vi "TriangleCache.vi"(4 "Point3D":T1, 6 "Rotation":T2, 8 "TriangleOperations":T4(ring), 9 "ScaleFac":sgl, 10 "ModelName":string, 11 "TrianglesIn":T3[](array[typedef])) -> (3 "TrianglesOut":T3[](array[typedef]))   [LabVIEW 2014]
uses:
  TypeDefs/TriangleFace.ctl
  TypeDefs/Point3D.ctl
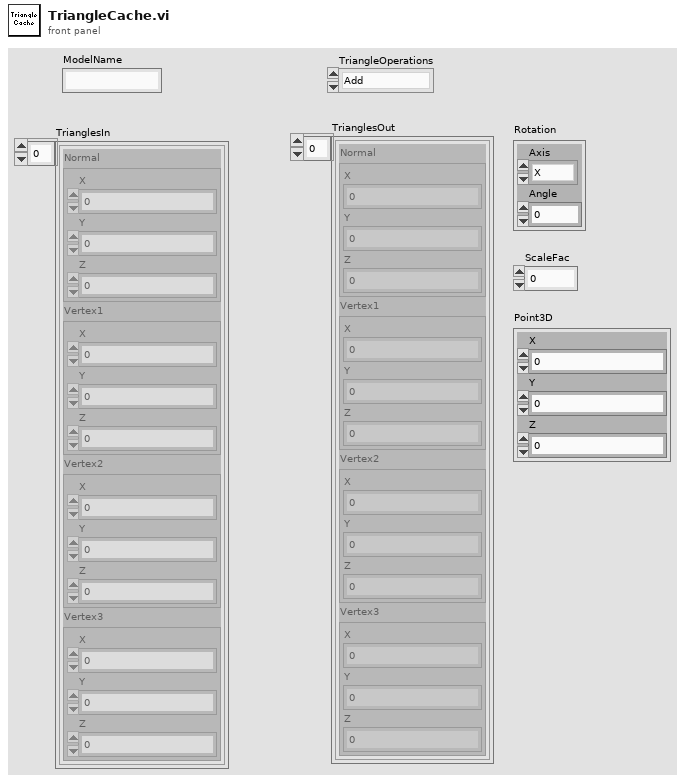
[diagram p1: front panel]
types:
  T1 = typedef "Point3D.ctl" = cluster{"X":sgl, "Y":sgl, "Z":sgl}
  T2 = cluster{"Axis":enum16{"X", "Y", "Z"}, "Angle":sgl}
  T3 = typedef "TriangleFace.ctl" = cluster{"Normal":T1, "Vertex1":T1, "Vertex2":T1, "Vertex3":T1}
  T4 = enum16{"Add", "Get", "Scale", "Rotate", "Translate", "Symmetry", "Clear"}
  T5 = cluster{"ModelName":string, "TrianglesOut":T3[]}[]
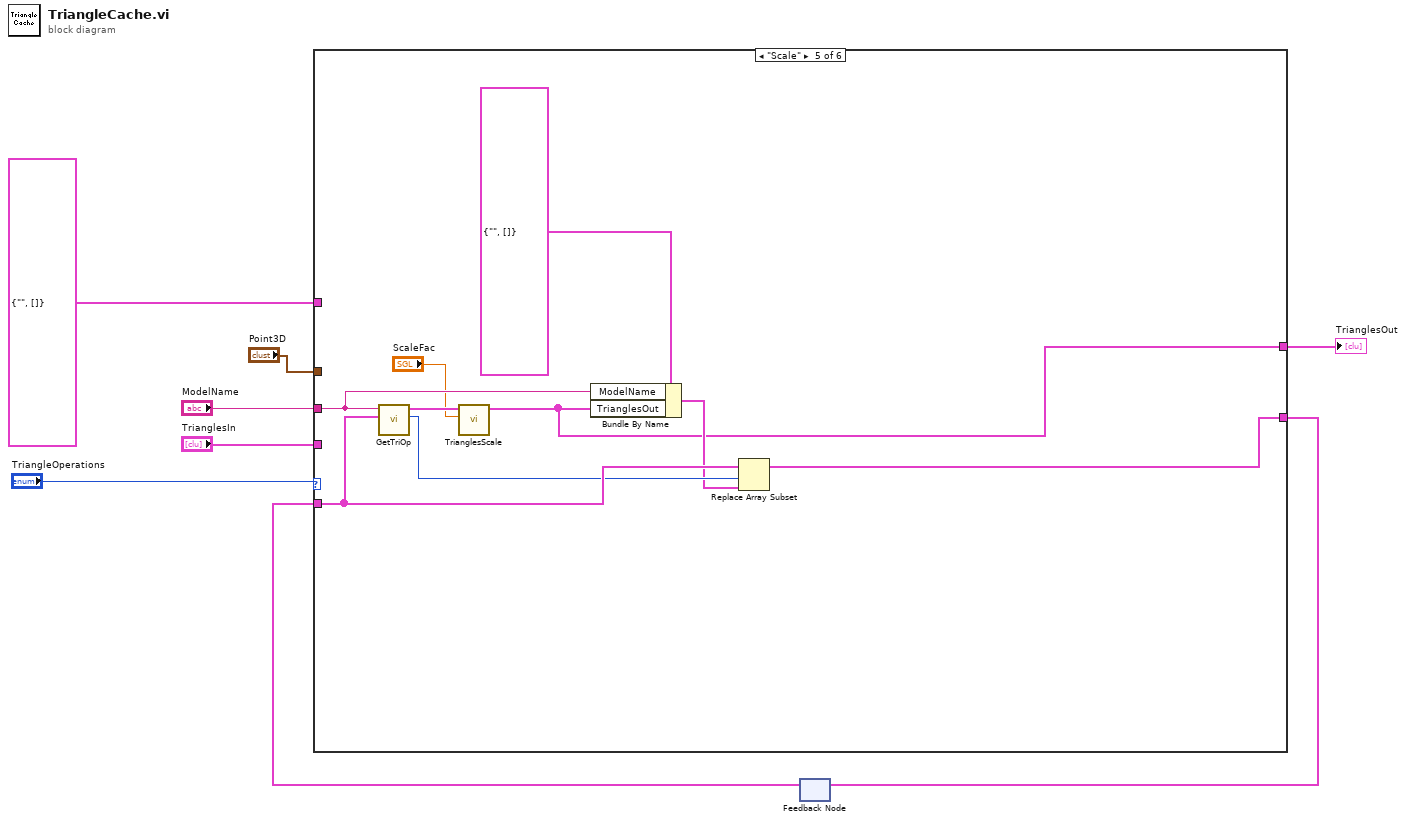
[diagram p0: block diagram]
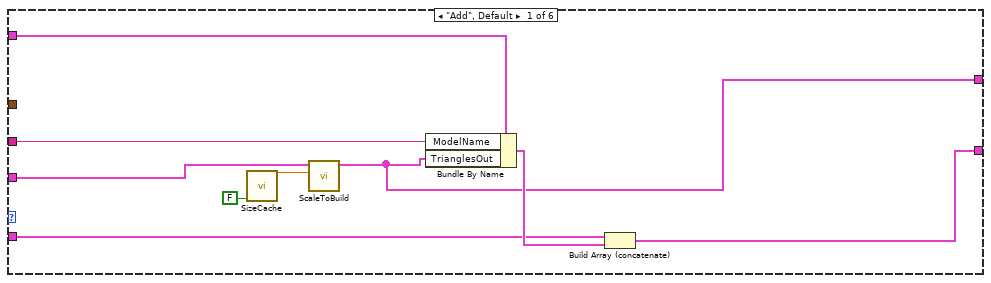
[diagram p2: hidden frame]
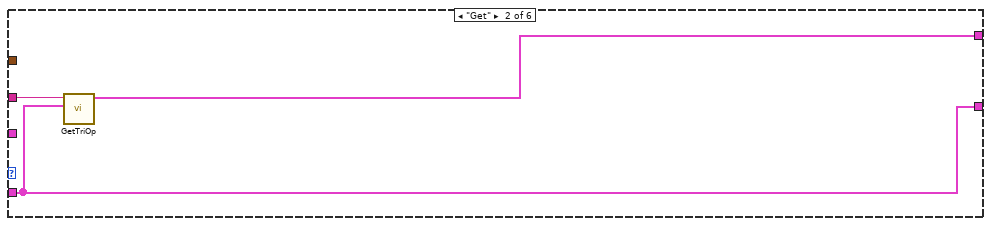
[diagram p3: hidden frame]
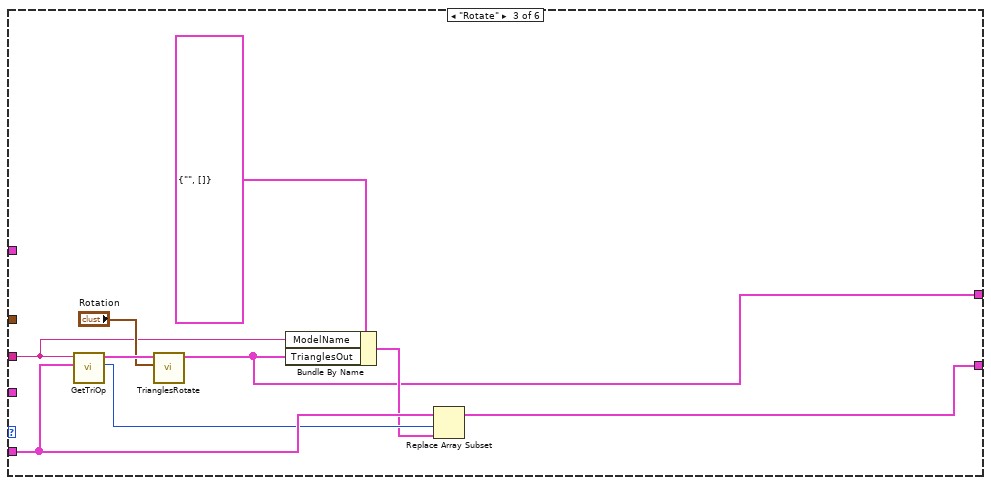
[diagram p4: hidden frame]
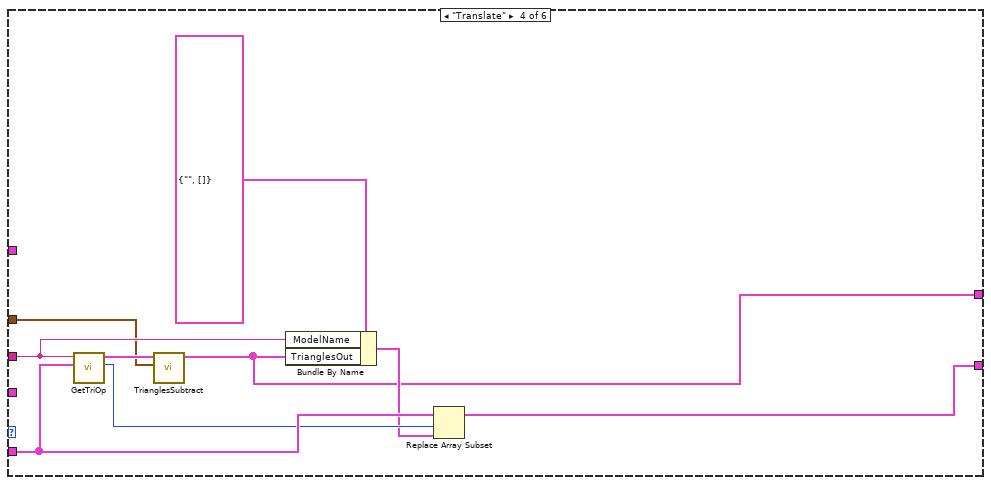
[diagram p5: hidden frame]
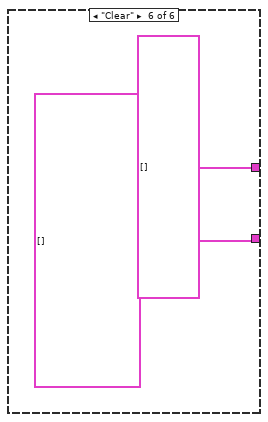
[diagram p6: hidden frame]
diagram:
  n1 = feedback #1() -> (w3:T5)  [unwired: 1 in]
  n2 = case shown="\"Scale\"" "TriangleOperations" {
    tunnel: cluster{"ModelName":string, "TrianglesOut":T3[]} {"ModelName"="", "TrianglesOut"=[]} ("Model") -> [w17 _ _ _ _ _]
    tunnel: "ModelName" -> [w16 w20 w24 w34 w43 _]
    tunnel: "TrianglesIn" -> [w10 _ _ _ _ _]
    tunnel: [w13 w18 w22 w32 w41 T5 []] -> w4
    tunnel: w3 -> [w14 w18 w27 w37 w46 _]
    tunnel: [w9 w19 w21 w31 w40 T3[] [] ("TrianglesOut")] -> w2
    tunnel: "Point3D" -> [_ _ _ w30 _ _]
    frame "Add", Default {
      n3 = call "SizeCache.vi"("Set"=FALSE) -> ("SizeOut"=w11:dbl)  [unwired: 10 in]
      n4 = call "ScaleToBuild.vi"("BuildSize"=w11, "Triangles"=w10) -> ("TrianglesOut"=w9:T3[])  [unwired: 9 in]
      n5 = Bundle By Name(cluster=w17, "ModelName"=w16, "TrianglesOut"=w9) -> (w15:cluster{"ModelName":string, "TrianglesOut":T3[]})
      n6 = Build Array (concatenate)(w14, w15) -> (w13:T5)
    }
    frame "Get" {
      n7 = call "GetTriOp.vi"("Array"=w18, "ModelName"=w20) -> ("TrianglesOut"=w19:T3[])  [unwired: 8 in, 1 out]
    }
    frame "Rotate" {
      n8 = call "GetTriOp.vi"("Array"=w27, "ModelName"=w24) -> ("Index"=w26:i32, "TrianglesOut"=w29:T3[])  [unwired: 8 in]
      n9 = call "TrianglesRotate.vi"("Rotation"="Rotation", "TrianglesIn"=w29) -> ("TrianglesOut"=w21:T3[])  [unwired: 9 in]
      n10 = Bundle By Name(cluster=cluster{"ModelName":string, "TrianglesOut":T3[]} {"ModelName"="", "TrianglesOut"=[]} ("Model"), "ModelName"=w24, "TrianglesOut"=w21) -> (w23:cluster{"ModelName":string, "TrianglesOut":T3[]})
      n11 = Replace Array Subset(array=w27, new element=w23, index=w26) -> (w22:T5)
    }
    frame "Translate" {
      n12 = call "GetTriOp.vi"("Array"=w37, "ModelName"=w34) -> ("Index"=w36:i32, "TrianglesOut"=w38:T3[])  [unwired: 8 in]
      n13 = call "TrianglesSubtract.vi"("Point3D"=w30, "TrianglesIn"=w38) -> ("TrianglesOut"=w31:T3[])  [unwired: 9 in]
      n14 = Bundle By Name(cluster=cluster{"ModelName":string, "TrianglesOut":T3[]} {"ModelName"="", "TrianglesOut"=[]} ("Model"), "ModelName"=w34, "TrianglesOut"=w31) -> (w33:cluster{"ModelName":string, "TrianglesOut":T3[]})
      n15 = Replace Array Subset(array=w37, new element=w33, index=w36) -> (w32:T5)
    }
    frame "Scale" {
      n16 = call "GetTriOp.vi"("Array"=w46, "ModelName"=w43) -> ("Index"=w45:i32, "TrianglesOut"=w47:T3[])  [unwired: 8 in]
      n17 = call "TrianglesScale.vi"("ScaleFac"="ScaleFac", "TrianglesIn"=w47) -> ("TrianglesOut"=w40:T3[])  [unwired: 9 in]
      n18 = Bundle By Name(cluster=cluster{"ModelName":string, "TrianglesOut":T3[]} {"ModelName"="", "TrianglesOut"=[]} ("Model"), "ModelName"=w43, "TrianglesOut"=w40) -> (w42:cluster{"ModelName":string, "TrianglesOut":T3[]})
      n19 = Replace Array Subset(array=w46, new element=w42, index=w45) -> (w41:T5)
    }
    frame "Clear" {
    }
  }
  "TrianglesOut" <- w2
  n20 = feedback-in #1(w4) -> ()
